vi "tx-rx-loopback.vi"(0 "USRP IP address":string="192.168.10.88", 1 "RFNoC Graph Settings":T2, 2 "Rx Settings":T1={"frequency"=2000000000.0, "rate"=1000000.0, "antenna"="RX1", "gain"=0.0} {"frequency" format="%#_6p"; "rate" format="%#_6p"}, 3 "Tx Settings":T1={"frequency"=2000000000.0, "rate"=1000000.0, "antenna"="TX/RX0", "gain"=0.0} {"frequency" format="%#_6p"; "rate" format="%#_6p"}, 5 "Iteration Count":i32=3000000, 11 "Python Version":string(combo)="3.10") -> (4 "Iterations":u32, 6 "Tx Errors":cluster{"Error":string, "Count":dbl}[](array[cluster])=[{"Error"="Unknown", "Count"=0.0}, {"Error"="Underflow", "Count"=0.0}, {"Error"="Sequence", "Count"=0.0}, {"Error"="Time", "Count"=0.0}, {"Error"="Underflow (Packet)", "Count"=0.0}, {"Error"="Sequence (Burst)", "Count"=0.0}, {"Error"="User Payload", "Count"=0.0}], 8 "Rx Errors":cluster{"Error":string, "Count":dbl}[](array[cluster])=[{"Error"="Unknown", "Count"=0.0}, {"Error"="Timeout", "Count"=0.0}, {"Error"="Late", "Count"=0.0}, {"Error"="Broken Chain", "Count"=0.0}, {"Error"="Out of Sequence", "Count"=0.0}, {"Error"="Overfow", "Count"=0.0}, {"Error"="Alignment", "Count"=0.0}, {"Error"="Bad Packet", "Count"=0.0}], 10 "Displayed Samples":u64 format="%.3p", 15 "Error":errorcluster)   [LabVIEW 2025]
doc: "This example shows how to set up a basic Tx/Rx loopback and stream data using RF Network-on-chip (RFNoC). It uses the UHD RFNoC API for Python to configure the USRP device, stream data from the LabVIEW host to the USRP transmitter, loop it back to the USRP receiver and transfer the data back to the LabVIEW host."
uses:
  <vilib>/ChannelSupport/Channel Abort Instructions.ctl
  <extravilib>/ChannelInstances/High Speed Stream-c(u32,u32,u64,u64,i32,u32,bool)/_Read For Replicate.vi
  <extravilib>/ChannelInstances/High Speed Stream-a[.,.](u64)/_Read For Replicate.vi
  <extravilib>/ChannelInstances/High Speed Stream-c(u32,u32,u64,u64,i32,u32,bool)/Instantiate.vi
  <extravilib>/ChannelInstances/High Speed Stream-a[.,.](u64)/Instantiate.vi
  <extravilib>/ChannelInstances/High Speed Stream-a[.,.](u64)/)Channel.vi
  <extravilib>/ChannelInstances/High Speed Stream-c(u32,u32,u64,u64,i32,u32,bool)/)Channel.vi
  <extravilib>/ChannelInstances/High Speed Stream-c(u32,u32,u64,u64,i32,u32,bool)/Abort Signal/Init Signal.vi
  <extravilib>/ChannelInstances/High Speed Stream-a[.,.](u64)/Abort Signal/Init Signal.vi
  <vilib>/measure/maspectr.llb/FFT Spectrum (Mag-Phase) for 1 Chan (CDB).vi
  <vilib>/measure/NI_MAPro.lvlib
  <extravilib>/ChannelInstances/High Speed Stream-a[.,.](u64).lvlib
  <vilib>/measure/NI_MABase.lvlib
  <extravilib>/ChannelInstances/High Speed Stream-c(u32,u32,u64,u64,i32,u32,bool).lvlib
panel:
  in  "Tone Amplitude":dbl=0.707
  in  "Tone Frequency (Hz)":dbl=10000.0 format="%#_6p"
  in  "Waveform Size":dbl=10000.0
  in  "Rx Graphs":T3(tab)
  out "Received Signal":waveform(sgl)[](graph)
  out "Rx Signal Magnitude":cluster{"f0":dbl, "df":dbl, "magnitude":dbl[]}(graph)
  in  "Title":string="LabVIEW - RFNoC Tx-Rx-Loopback Example"
  in  "Counters":enum32{"", "Debug Panel"}(tab)
  out "Sent Samples":u64 format="%.3p"
  out "Received Samples":u64 format="%.3p"
  out "Duration":u32
  out "Runtime":dbl
  out "Tx Waveform Graph":waveform(dbl)[](graph)
  in  "Stop":bool
  # "(set -1 for infinite)"
  # "Note: antenna names might differ between USRP device types. Here, settings for an X410 device are preset."
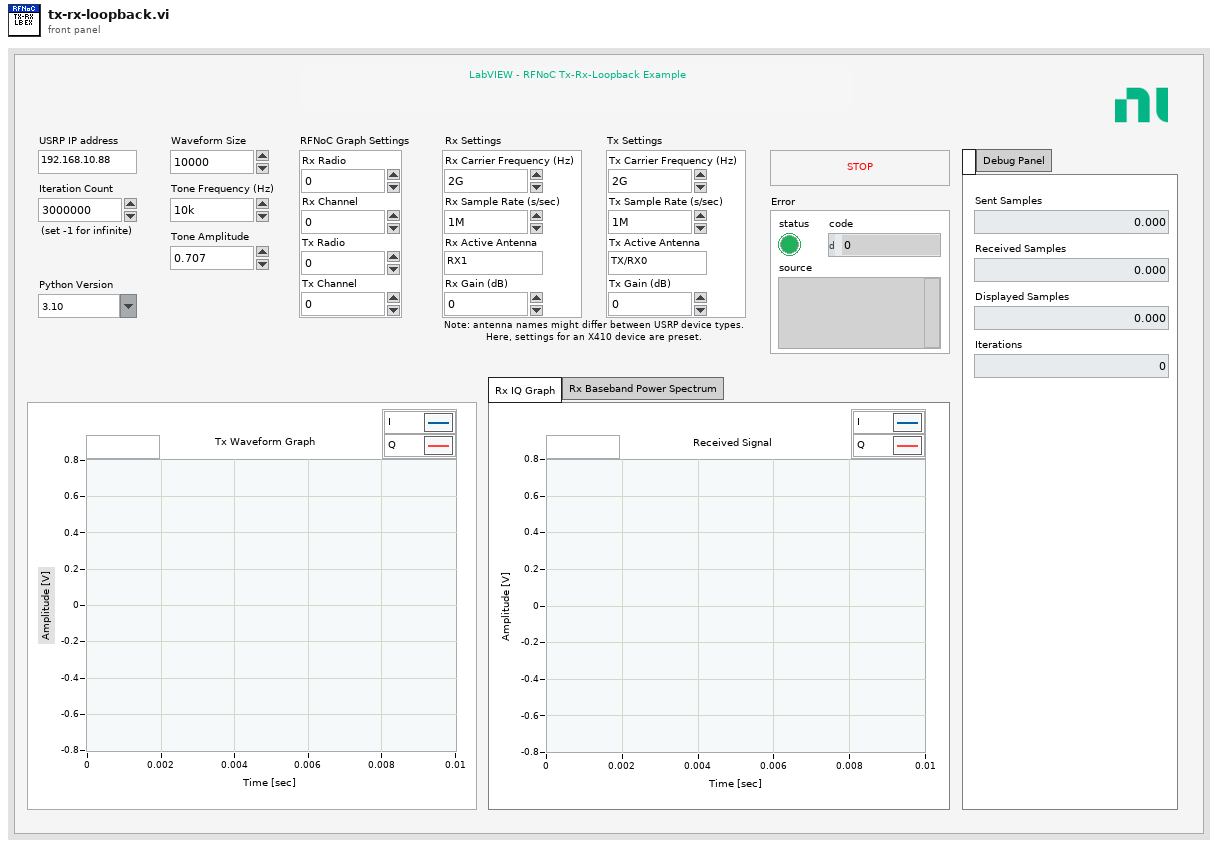
[diagram p1: front panel]
types:
  T1 = cluster{"frequency":dbl, "rate":dbl, "antenna":string, "gain":dbl}
  T2 = cluster{"rx_radio":u32, "rx_chan":u32, "tx_radio":u32, "tx_chan":u32}
  T3 = enum32{"Rx IQ Graph", "Rx Baseband Power Spectrum"}
  T4 = cluster{"dB On (F)":bool, "unwrap phase (F)":bool, "convert to degree (F)":bool}
  T5 = cluster{"Iterations":u32, "Duration":u32, "Sent Samples":u64, "Received Samples":u64, "Rx Error":i32, "Tx Error":u32, "Out of Sequence":bool}
  T6 = typedef "Channel Abort Instructions.ctl" = enum16{"No abort", "Abort now", "Abort if timeout"}
  T7 = cluster{"Rx Error":i32, "Out of Sequence":bool, "Received":i32}
  T8 = typedef "High Speed Stream-c(u32,u32,u64,u64,i32,u32,bool).lvlib/)Channel.ctl" = refnum<queue>
  T9 = typedef "High Speed Stream-a[.,.](u64).lvlib/)Channel.ctl" = refnum<queue>
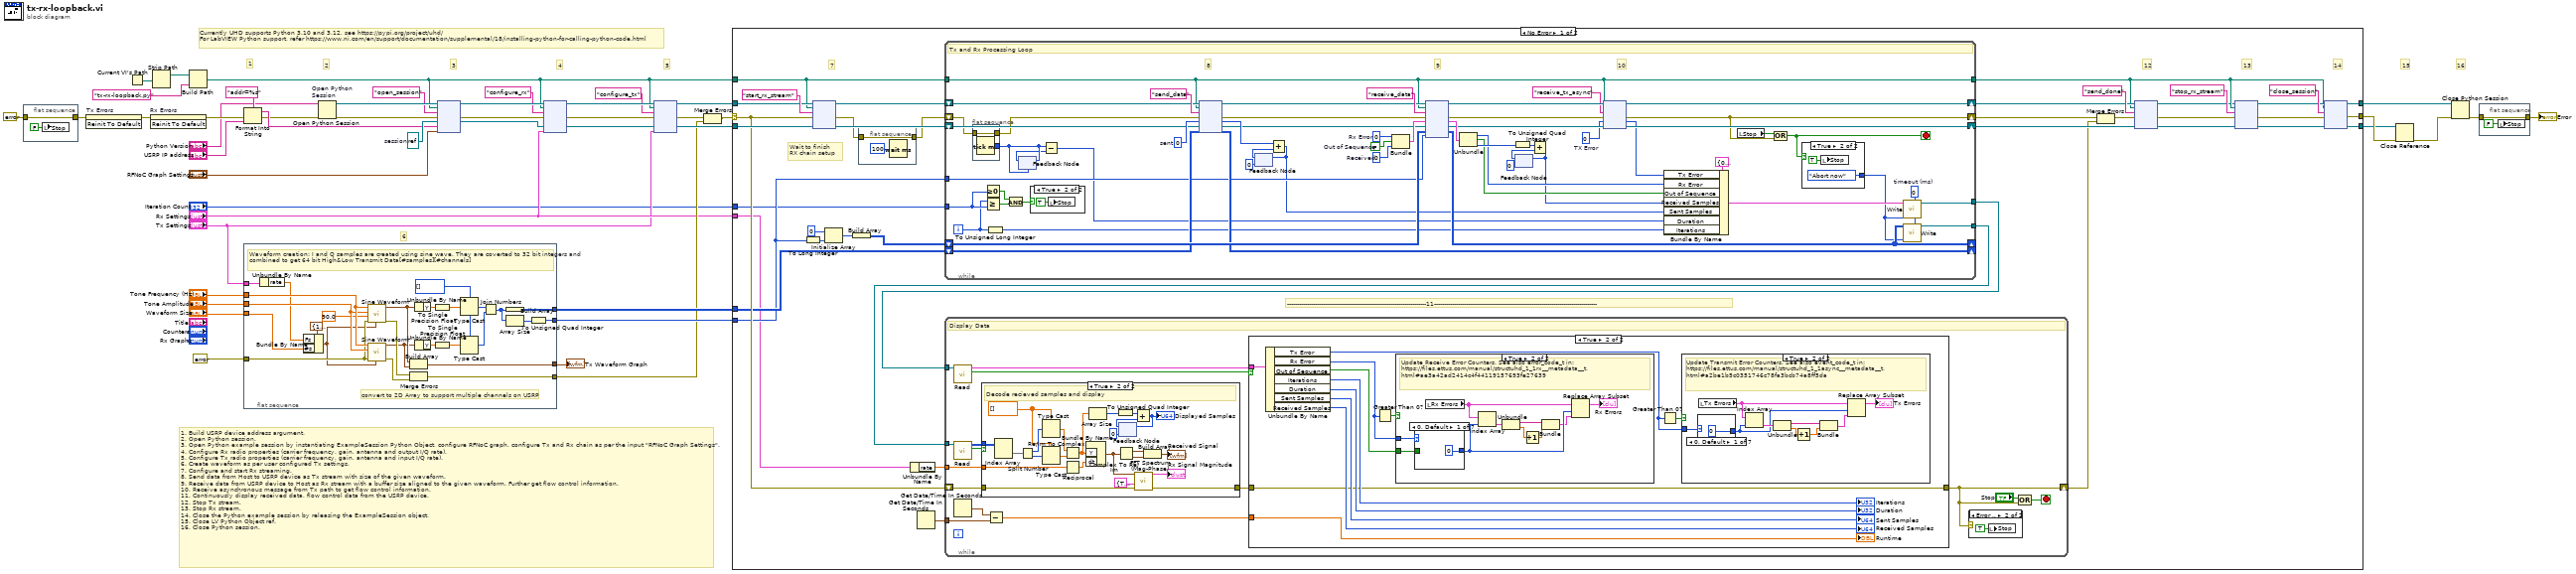
[diagram p0: block diagram]
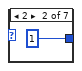
[diagram p4: hidden frame]
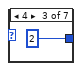
[diagram p5: hidden frame]
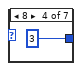
[diagram p6: hidden frame]
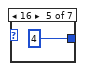
[diagram p7: hidden frame]
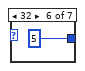
[diagram p8: hidden frame]
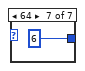
[diagram p9: hidden frame]
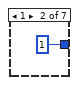
[diagram p11: hidden frame]
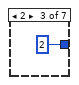
[diagram p12: hidden frame]
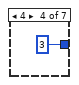
[diagram p13: hidden frame]
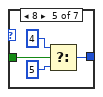
[diagram p14: hidden frame]
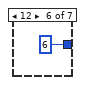
[diagram p15: hidden frame]
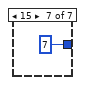
[diagram p16: hidden frame]
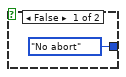
[diagram p20: hidden frame]
diagram:
  w42 = refnum<k38> refnum  # session
  # "Currently UHD supports Python 3.10 and 3.12, see https://pypi.org/project/uhd/\nFor LabVIEW Python support, refer https://www.ni.com/en/support/documentation/supplemental/18/installing-python-for-calling-python-code.html"
  # "1. Build USRP device address argument.\n2. Open Python session.\n3. Open Python example session by instantiating ExampleSession Python Object, configure RFNoC graph, configure Tx and Rx chain as per the input \"RFNoC Graph Settings\".\n4. Configure Rx radio properties (carrier frequency, gain, antenna and output I/Q rate).\n5. Configure Tx radio properties (carrier frequency, gain, antenna and input I/Q rate).\n6. Create waveform as per user configured Tx settings.\n7. Configure and start Rx streaming.\n8. Send data from Host to USRP device as Tx stream with size of the given waveform.\n9. Receive data from USRP device to Host as Rx stream with a buffer size aligned to the given waveform. Further get flow control information.\n10. Receive asynchronous message from Tx path to get flow control information.\n11. Continuously display received data, flow control data from the USRP device.\n12. Stop Tx stream.\n13. Stop Rx stream.\n14. Close the Python example session by releasing the ExampleSession object.\n15. Close LV Python Object ref.\n16. Close Python session."
  # "16"
  # "15"
  # "6"
  # "5"
  # "4"
  # "3"
  # "2"
  # "1"
  n1 = flat-sequence {
    tunnel: errorcluster {"status"=FALSE, "code"=0, "source"=""} ("error constant") -> [w49]
    tunnel: [w49] -> w10
    frame #0 {
      n2 = local write "Stop"(FALSE ("Stop")) -> ()
    }
  }
  n3 = invoke on="Tx Errors" class="Arr (strict)" method="Reinit To Default"(error in=w10) -> (error out=w28:errorcluster)  [unwired: 2 in, 2 out]
  n4 = Current VI's Path() -> (path=w41:path)
  n5 = invoke on="Rx Errors" class="Arr (strict)" method="Reinit To Default"(error in=w28) -> (error out=w24:errorcluster)  [unwired: 2 in, 2 out]
  n6 = Strip Path(path=w41) -> (stripped path=w40:path)  [unwired: 1 out]
  n7 = Build Path(base path=w40, name or relative path="tx-rx-loopback.py") -> (appended path=w29:path)
  n8 = Format Into String(format string="addr=%s", error in=w24, "USRP IP address") -> (resulting string=w37:string, error out=w23:errorcluster)  [unwired: 1 in]
  n9 = flat-sequence {
    tunnel: "Tone Frequency (Hz)" -> [w75]
    tunnel: "Tone Amplitude" -> [w74]
    tunnel: "Waveform Size" -> [w73]
    tunnel: [w72] -> w17
    tunnel: [w71] -> w16
    tunnel: [w70] -> w15
    tunnel: [w69] -> w14
    tunnel: errorcluster {"status"=FALSE, "code"=0, "source"=""} ("error in") -> [w68]
    tunnel: "Tx Settings" -> [w51]
    frame #0 {
      w64 = u32[] [] ("element")
      # "convert to 2D Array to support multiple channels on USRP"
      # "Waveform creation: I and Q samples are created using sine wave. They are coverted to 32 bit integers and combined to get 64 bit High&Low Transmit Data[#samples][#channels]"
      n10 = Unbundle By Name(w51) -> ("rate"=w50:dbl)
      n11 = Bundle By Name(cluster=cluster{"Fs":dbl, "#s":dbl} {"Fs"=1000.0, "#s"=1000.0} ("sampling info"), "Fs"=w50, "#s"=w73) -> (w66:cluster{"Fs":dbl, "#s":dbl})
      n12 = call <vilib>:"Sine Waveform.vi"("sampling info"=w66, "error in (no error)"=w68, "phase"=90.0, "amplitude"=w74, "frequency"=w75) -> ("error out"=w55:errorcluster, "signal out"=w53:waveform(dbl))  [unwired: 5 in]
      n13 = call <vilib>:"Sine Waveform.vi"("sampling info"=w66, "error in (no error)"=w68, "amplitude"=w74, "frequency"=w75) -> ("error out"=w54:errorcluster, "signal out"=w52:waveform(dbl))  [unwired: 6 in]
      n14 = Build Array(w53, w52) -> (w69:waveform(dbl)[])
      n15 = Merge Errors(w55, w54) -> (w70:errorcluster)
      n16 = Unbundle By Name ("Get Waveform Components")(w53) -> ("Y"=w58:dbl[])
      n17 = Unbundle By Name ("Get Waveform Components")(w52) -> ("Y"=w60:dbl[])
      n18 = To Single Precision Float(number=w58) -> (single precision float=w57:sgl[])
      n19 = To Single Precision Float(number=w60) -> (single precision float=w59:sgl[])
      n20 = Type Cast(type=w64, x=w57) -> (*(type *) &x=w62:u32[])
      n21 = Type Cast(type=w64, x=w59) -> (*(type *) &x=w61:u32[])
      n22 = Join Numbers(hi=w62, lo=w61) -> ((hi.lo)=w63:u64[])
      n23 = Build Array(w63) -> (w72:u64[][])
      n24 = Array Size(array=w63) -> (size(s)=w56:i32)
      n25 = To Unsigned Quad Integer(1:w56) -> (0:w71:u64)
    }
  }
  n26 = Open Python Session "Open Python\nSession"(python version="Python Version", 3:w23) -> (session out=w47:refnum<k35>, error out=w25:errorcluster)  [unwired: 1 in]
  n27 = node ("Python Node")(w47, w29, "open_session" ("function name"), w25, w42, w37, "RFNoC Graph Settings") -> (w44:refnum<k35>, w45:errorcluster, w13:refnum<k38>)  [unwired: 2 in, 2 out]
  n28 = node ("Python Node")(w44, w29, "configure_rx" ("function name"), w45, w13, "Rx Settings") -> (w32:refnum<k35>, w26:errorcluster, w30:refnum<k38>)  [unwired: 3 in, 2 out]
  n29 = node ("Python Node")(w32, w29, "configure_tx" ("function name"), w26, w30, "Tx Settings") -> (w20:refnum<k35>, w18:errorcluster, w22:refnum<k38>)  [unwired: 3 in, 2 out]
  n30 = Merge Errors(w18, w15) -> (w21:errorcluster)
  n31 = case shown="No Error" w21 {
    selector: w21 -> [w91 w272]
    tunnel: [w112 w272] -> w36
    tunnel: [w110 w270] -> w35
    tunnel: [w108 w271] -> w34
    tunnel: w17 -> [w85 _]
    tunnel: w16 -> [w81 _]
    tunnel: w22 -> [w93 w271]
    tunnel: w20 -> [w95 w270]
    tunnel: w29 -> [w94 _]
    tunnel: "Rx Settings" -> [w80 _]
    tunnel: "Iteration Count" -> [w77 _]
    frame No Error {
      # "7"
      # "----------------------------------------------------------------------11----------------------------------------------------------------------------------"
      # "Wait to finish\nRX chain setup"
      # "14"
      # "13"
      # "12"
      n32 = To Long Integer(number=w81) -> (32bit integer=w100:i32)
      n33 = node ("Python Node")(w95, w94, "start_rx_stream" ("function name"), w91, w93) -> (w90:refnum<k35>, w79:errorcluster, w92:refnum<k38>)  [unwired: 2 in, 2 out]
      n34 = Initialize Array(u64 0 ("element"), w100) -> (w101:u64[])
      n35 = Build Array(w101) -> (w98:u64[][])
      n36 = flat-sequence {
        tunnel: w79 -> [w115]
        tunnel: [w115] -> w78
        frame #0 {
          n37 = Wait (ms)(milliseconds to wait=u32 100) -> ()  [unwired: 1 out]
        }
      }
      n38 = Unbundle By Name(w80) -> ("rate"=w97:dbl)
      n39 = Get Date/Time In Seconds() -> (seconds since 1Jan1904=w82:timestamp)
      n40 = while {
        tunnel: w94 -> [w238]
        shift-right: [w235] -> w83
        shift-left: w78 -> [w225]
        tunnel: [w238] -> w88
        shift-right: [w240] -> w86
        shift-left: w92 -> [w245]
        shift-right: [w236] -> w89
        shift-left: w90 -> [w247]
        shift-right: [w255] -> _
        shift-left: w98 -> [w258]
        tunnel: w81 -> [w232]
        tunnel: [w254] -> w106
        shift-right: [w242] -> _
        shift-left: w85 -> [w243]
        tunnel: w77 -> [w228]
        tunnel: [w210] -> w76
        i -> [w207]
        stop <- w217 stop-if-true
        w209 = FALSE  # Out of Sequence
        w229 = u32 0  # TX Error
        w211 = 0  # timeout (ms)
        w250 = u64 0  # sent
        w257 = 0  # Rx Error
        w256 = 0  # Received
        # "10"
        # "9"
        # "8"
        # "Tx and Rx Processing Loop"
        n41 = flat-sequence {
          tunnel: [w266] -> w226
          tunnel: w225 -> [w265]
          tunnel: [w265] -> w224
          frame #0 {
            n42 = Tick Count (ms)() -> (millisecond timer value=w266:u32)
          }
        }
        n43 = Greater Or Equal To 0?(x=w228) -> (x >= 0?=w231:bool)
        n44 = Greater Or Equal?(x=w207, y=w228) -> (x >= y?=w216:bool)
        n45 = To Unsigned Long Integer(number=w207) -> (unsigned 32bit integer=w206:u32)
        n46 = And(x=w231, y=w216) -> (x .and. y?=w208:bool)
        n47 = feedback #1(w226) -> (w215:u32)
        n48 = feedback-in #1(w226) -> ()
        n49 = case shown="True" w208 {
          frame False {
          }
          frame True {
            n50 = local write "Stop"(TRUE ("Stop")) -> ()
          }
        }
        n51 = Subtract(x=w226, y=w215) -> (x-y=w218:u32)
        n52 = node ("Python Node")(w247, w238, "send_data" ("function name"), w224, w250, w245, w243) -> (w248:refnum<k35>, w246:errorcluster, w249:u64, w244:refnum<k38>, w242:u64[][])  [unwired: 2 out]
        n53 = feedback #2(u64 0) -> (w252:u64)
        n54 = Add(x=w249, y=w252) -> (x+y=w219:u64)
        n55 = feedback-in #2(w219) -> ()
        n56 = Bundle("Rx Error"=w257, "Out of Sequence"=w209, "Received"=w256) -> (w262:T7)  [unwired: 1 in]
        n57 = node ("Python Node")(w248, w238, "receive_data" ("function name"), w246, w262, w244, w258, w232) -> (w237:refnum<k35>, w239:errorcluster, w261:T7, w241:refnum<k38>, w255:u64[][])  [unwired: 1 in, 2 out]
        n58 = Unbundle(w261) -> ("Rx Error"=w222:i32, "Out of Sequence"=w221:bool, "Received"=w233:i32)
        n59 = To Unsigned Quad Integer(1:w233) -> (0:w234:u64)
        n60 = feedback #3(u64 0) -> (w260:u64)
        n61 = Add(x=w234, y=w260) -> (x+y=w220:u64)
        n62 = feedback-in #3(w220) -> ()
        n63 = node ("Python Node")(w237, w238, "receive_tx_async" ("function name"), w239, w229, w241) -> (w236:refnum<k35>, w235:errorcluster, w223:u32, w240:refnum<k38>)  [unwired: 2 out]
        n64 = Bundle By Name(cluster=T5 {"Iterations"=0, "Duration"=0, "Sent Samples"=0, "Received Samples"=0, "Rx Error"=0, "Tx Error"=0, "Out of Sequence"=FALSE} ("input cluster"), "Tx Error"=w223, "Rx Error"=w222, "Out of Sequence"=w221, "Received Samples"=w220, "Sent Samples"=w219, "Duration"=w218, "Iterations"=w206) -> (w213:T5)
        n65 = local read "Stop"() -> (w227:bool)
        n66 = Compound Arithmetic op=OR(w227, w235) -> (w217:bool)
        n67 = case shown="True" w217 {
          tunnel: [Channel_Abort_Instructions."No abort" ("abort status (no abort)") Channel_Abort_Instructions."Abort now" ("abort status (no abort)")] -> w212
          frame False {
          }
          frame True {
            n68 = local write "Stop"(TRUE ("Stop")) -> ()
          }
        }
        n69 = call <extravilib>:"Write.vi"("timeout in ms (-1)"=w211, "abort status (no abort)"=w212, "element"=w213) -> ("channel"=w210:T8)  [unwired: 6 in, 2 out]
        n70 = call <extravilib>:"Write.vi"("timeout in ms (-1)"=w211, "abort status (no abort)"=w212, "element"=w255) -> ("channel"=w254:T9)  [unwired: 6 in, 2 out]
      }
      n71 = while {
        tunnel: w97 -> [w131]
        shift-right: [w117] -> w84
        shift-left: w91 -> [w130]
        tunnel: w106 -> [w129]
        tunnel: w82 -> [w124]
        tunnel: w76 -> [w121]
        stop <- w126 stop-if-true
        # "Display Data"
        n72 = call <extravilib>:"Read.vi"("channel"=w121) -> ("element valid?"=w119:bool, "element"=w120:T5)  [unwired: 6 in, 3 out]
        n73 = call <extravilib>:"Read.vi"("channel"=w129) -> ("element valid?"=w127:bool, "element"=w128:u64[][])  [unwired: 6 in, 3 out]
        n74 = Get Date/Time In Seconds() -> (seconds since 1Jan1904=w125:timestamp)
        n75 = case shown="True" w127 {
          tunnel: w128 -> [_ w201]
          tunnel: w131 -> [_ w193]
          tunnel: [w181 w190] -> w118
          tunnel: w130 -> [w181 w189]
          frame False {
          }
          frame True {
            w202 = sgl[] [] ("single precision float")
            # "Decode recieved samples and display"
            n76 = Index Array(array=w201) -> (element=w184:u64[])  [unwired: 2 in]
            n77 = Split Number(x=w184) -> (hi(x)=w203:u32[], lo(x)=w204:u32[])
            n78 = Type Cast(type=w202, x=w203) -> (*(type *) &x=w195:sgl[])
            n79 = Type Cast(type=w202, x=w204) -> (*(type *) &x=w194:sgl[])
            n80 = Re/Im To Complex(1:w194, 2:w195) -> (0:w185:csg[])
            n81 = Reciprocal(x=w193) -> (1/x=w191:dbl)
            n82 = Bundle By Name ("Build Waveform")("Y"=w185, "dt"=w191) -> (w196:waveform(csg))  [unwired: 1 in]
            n83 = Array Size(array=w185) -> (size(s)=w183:i32)
            n84 = To Unsigned Quad Integer(1:w183) -> (0:w182:u64)
            n85 = Complex To Re/Im(x + iy=w196) -> (x=w198:waveform(sgl), y=w197:waveform(sgl))
            n86 = feedback #4(u64 0) -> (w186:u64)
            n87 = Add(x=w182, y=w186) -> (x+y=w187:u64)
            "Displayed Samples" <- w187
            n88 = feedback-in #4(w187) -> ()
            n89 = call-poly <vilib>:"FFT Spectrum (Mag-Phase).vi"("error in (no error)"=w189, "view"=T4 {"dB On (F)"=TRUE, "unwrap phase (F)"=FALSE, "convert to degree (F)"=FALSE}, "time signal"=w196) -> ("error out"=w190:errorcluster, "magnitude"=→"Rx Signal Magnitude":cluster{"f0":dbl, "df":dbl, "magnitude":dbl[]})  [unwired: 4 in, 3 out]
            n90 = Build Array(w198, w197) -> (→"Received Signal":waveform(sgl)[])
          }
        }
        n91 = Subtract(x=w125, y=w124) -> (x-y=w123:dbl)
        n92 = case shown="True" w119 {
          tunnel: w123 -> [_ w144]
          tunnel: w120 -> [_ w137]
          tunnel: w118 -> [w132 w133]
          tunnel: [w132 w133] -> w117
          frame False {
          }
          frame True {
            n93 = Unbundle By Name(w137) -> ("Tx Error"=w142:u32, "Rx Error"=w143:i32, "Out of Sequence"=w136:bool, "Iterations"=→"Iterations":u32, "Duration"=→"Duration":u32, "Sent Samples"=→"Sent Samples":u64, "Received Samples"=→"Received Samples":u64)
            n94 = Greater Than 0?(x=w143) -> (x > 0?=w135:bool)
            n95 = case shown="True" w135 {
              tunnel: w143 -> [_ w170]
              tunnel: w136 -> [_ w168]
              frame False {
              }
              frame True {
                # "Update Receive Error Counters. See also error_code_t in: \nhttps://files.ettus.com/manual/structuhd_1_1rx__metadata__t.html#ae3a42ad2414c4f44119157693fe27639"
                n96 = case shown="0, Default" w170 {
                  tunnel: [0 ("error_code") 1 ("error_code") 2 ("error_code") 3 ("error_code") w175 6 ("error_code") 7 ("error_code")] -> w169
                  tunnel: w168 -> [_ _ _ _ w178 _ _]
                  frame 0, Default {
                  }
                  frame 1 {
                  }
                  frame 2 {
                  }
                  frame 4 {
                  }
                  frame 8 {
                    n97 = Select(t=4 ("error_code"), s=w178, f=5 ("error_code")) -> (s? t:f=w175:i32)
                  }
                  frame 12 {
                  }
                  frame 15 {
                  }
                }
                n98 = local read "Rx Errors"() -> (w162:cluster{"Error":string, "Count":dbl}[])
                n99 = Index Array(array=w162, index=w169) -> (element=w167:cluster{"Error":string, "Count":dbl})
                n100 = Unbundle(w167) -> ("Error"=w166:string, "Count"=w165:dbl)
                n101 = Increment(x=w165) -> (x+1=w164:dbl)
                n102 = Bundle("Error"=w166, w164) -> (w163:cluster{"Error":string, dbl})  [unwired: 1 in]
                n103 = Replace Array Subset(array=w162, new element=w163, index=w169) -> (→"Rx Errors":cluster{"Error":string, "Count":dbl}[])
              }
            }
            n104 = Greater Than 0?(x=w142) -> (x > 0?=w134:bool)
            n105 = case shown="True" w134 {
              tunnel: w142 -> [_ w153]
              frame False {
              }
              frame True {
                # "Update Transmit Error Counters. See also event_code_t in:\nhttps://files.ettus.com/manual/structuhd_1_1async__metadata__t.html#a2be1b5c0351746c78fa3bcb74a8ff5da"
                n106 = case shown="0, Default" w153 {
                  tunnel: [0 ("unsigned 64bit integer") 1 ("unsigned 64bit integer") 2 ("unsigned 64bit integer") 3 ("unsigned 64bit integer") 4 ("unsigned 64bit integer") 5 ("unsigned 64bit integer") 6 ("unsigned 64bit integer")] -> w148
                  frame 0, Default {
                  }
                  frame 2 {
                  }
                  frame 4 {
                  }
                  frame 8 {
                  }
                  frame 16 {
                  }
                  frame 32 {
                  }
                  frame 64 {
                  }
                }
                n107 = local read "Tx Errors"() -> (w146:cluster{"Error":string, "Count":dbl}[])
                n108 = Index Array(array=w146, index=w148) -> (element=w149:cluster{"Error":string, "Count":dbl})
                n109 = Unbundle(w149) -> ("Error"=w151:string, "Count"=w152:dbl)
                n110 = Increment(x=w152) -> (x+1=w150:dbl)
                n111 = Bundle("Error"=w151, w150) -> (w147:cluster{"Error":string, dbl})  [unwired: 1 in]
                n112 = Replace Array Subset(array=w146, new element=w147, index=w148) -> (→"Tx Errors":cluster{"Error":string, "Count":dbl}[])
              }
            }
            "Runtime" <- w144
          }
        }
        n113 = case shown="Error .." w117 {
          frame No Error {
          }
          frame Error {
            n114 = local write "Stop"(TRUE ("Stop")) -> ()
          }
        }
        n115 = Compound Arithmetic op=OR("Stop", w117) -> (w126:bool)
      }
      n116 = Merge Errors(w83, w84) -> (w104:errorcluster)
      n117 = node ("Python Node")(w89, w88, "send_done" ("function name"), w104, w86) -> (w87:refnum<k35>, w103:errorcluster, w105:refnum<k38>)  [unwired: 2 in, 2 out]
      n118 = node ("Python Node")(w87, w88, "stop_rx_stream" ("function name"), w103, w105) -> (w111:refnum<k35>, w102:errorcluster, w109:refnum<k38>)  [unwired: 2 in, 2 out]
      n119 = node ("Python Node")(w111, w88, "close_session" ("function name"), w102, w109) -> (w110:refnum<k35>, w112:errorcluster, w108:refnum<k38>)  [unwired: 2 in, 2 out]
    }
    frame Error {
    }
  }
  n120 = Close Reference(reference=w34, error in (no error)=w36) -> (error out=w33:errorcluster)
  n121 = Close Python Session(session in=w35, error in=w33) -> (11:w31:errorcluster)
  n122 = flat-sequence {
    tunnel: [w273] -> w27
    tunnel: w31 -> [w273]
    frame #0 {
      n123 = local write "Stop"(FALSE ("Stop")) -> ()
    }
  }
  "Error" <- w27
  "Tx Waveform Graph" <- w14
